vi "Benchmark exprParser.vi"() -> ()   [LabVIEW 2015]
panel:
  in  "Iterations":i32=1000000
  out "dt":u32
  out "y":dbl[](array[numeric])
  out "x":dbl[](array[numeric])
  in  "szExpr":string="1*x^2+2*x+2"
  out "error out":errorcluster
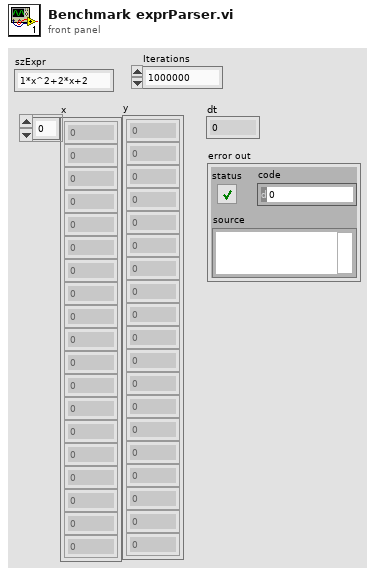
[diagram p1: front panel]
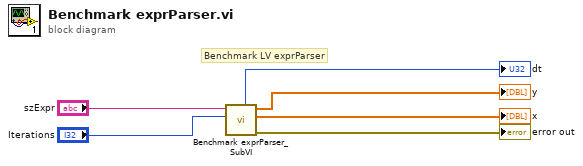
[diagram p0: block diagram]
diagram:
  # "Benchmark LV exprParser"
  n1 = call "Benchmark exprParser_SubVI.vi"("Iterations"="Iterations", "Expression"="szExpr") -> ("error out"=→"error out":errorcluster, "x"=→"x":dbl[], "y"=→"y":dbl[], "dt"=→"dt":u32)  [unwired: 6 in]
